vi "SMTP Email Send Message Charset.vi"(0 "recipients":string[](array[string]), 1 "mail server":string, 2 "return address":string, 3 "character set (us-ascii)":string="us-ascii", 5 "subject ([No Subject])":string="[No Subject]", 7 "message":string, 11 "error in (no error)":errorcluster, 12 "username":string, 13 "password":string, 14 "translit":string="MacRoman iso-8859-1 macroman.trl, ToUpper iso-8859-1 toupper.trl,\nMacRomanUp MacRoman toupper.trl") -> (4 "invalid recipients":string[](array[string]), 15 "error out":errorcluster)   [LabVIEW 2012, in "NewNI_SMTPEmail.lvlib"]
doc: "Sends a text email to a list of recipients."
uses:
  NewNI_SMTPEmail.lvlib
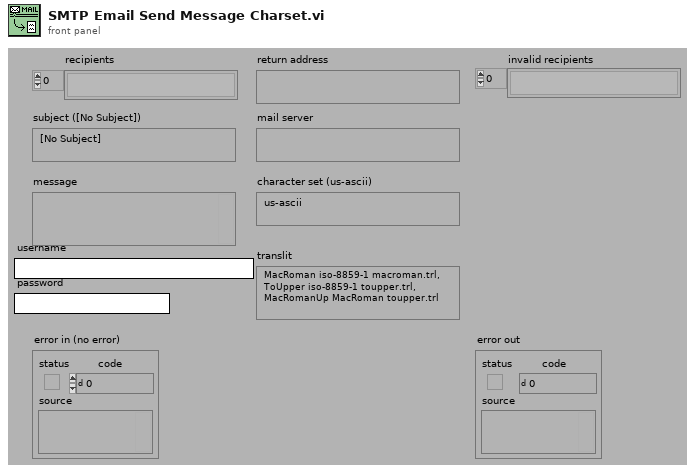
[diagram p1: front panel]
types:
  T1 = typedef "NewNI_SMTPEmail.lvlib/SMTP Email Session.ctl" = refnum<k1>
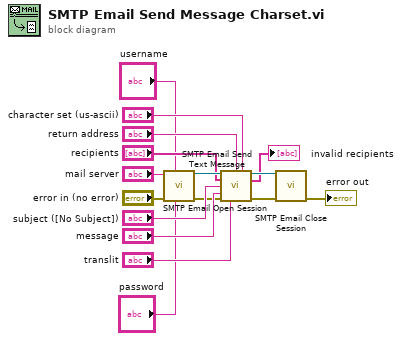
[diagram p0: block diagram]
diagram:
  n1 = call "SMTP Email Open Session.vi"("password"="password", "username"="username", "error in (no error)"="error in (no error)", "mail server"="mail server") -> ("error out"=w4:errorcluster, "smtp session out"=w13:T1)  [unwired: 1 in, 4 out]
  n2 = call "SMTP Email Send Text Message.vi"("smtp session"=w13, "return address"="return address", "character set"="character set (us-ascii)", "recipients"="recipients", "subject"="subject ([No Subject])", "message"="message", "error in (no error)"=w4, "translit"="translit") -> ("smtp session out"=w11:T1, "invalid recipients"=→"invalid recipients":string[], "error out"=w12:errorcluster)  [unwired: 5 out]
  n3 = call "SMTP Email Close Session.vi"("error in (no error)"=w12, "smtp session"=w11) -> ("error out"=→"error out":errorcluster)  [unwired: 1 in, 4 out]
